vi "loadDTCs.vi"(10 "DTCs":T1[](array[typedef])) -> (2 "dtcs":string[](array[string]))   [LabVIEW 2018]
uses:
  <vilib>/Automotive Diagnostic Command Set/Diagnostic Protocols.llb/Diagnostic Trouble Code.ctl
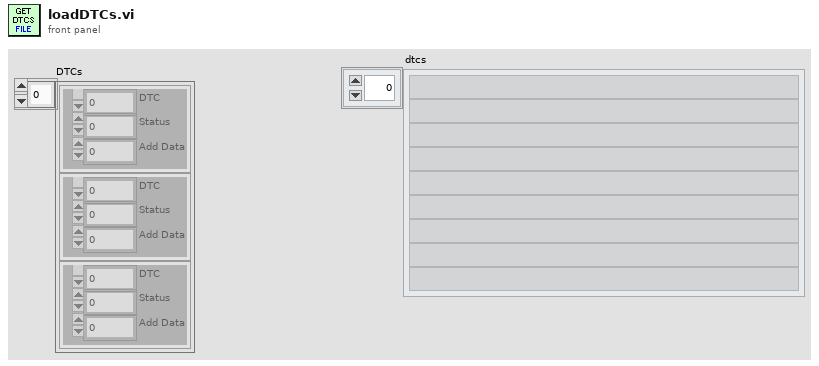
[diagram p1: front panel]
types:
  T1 = typedef "Diagnostic Trouble Code.ctl" = cluster{"DTC":u32, "Status":u32, "Add Data":u32}
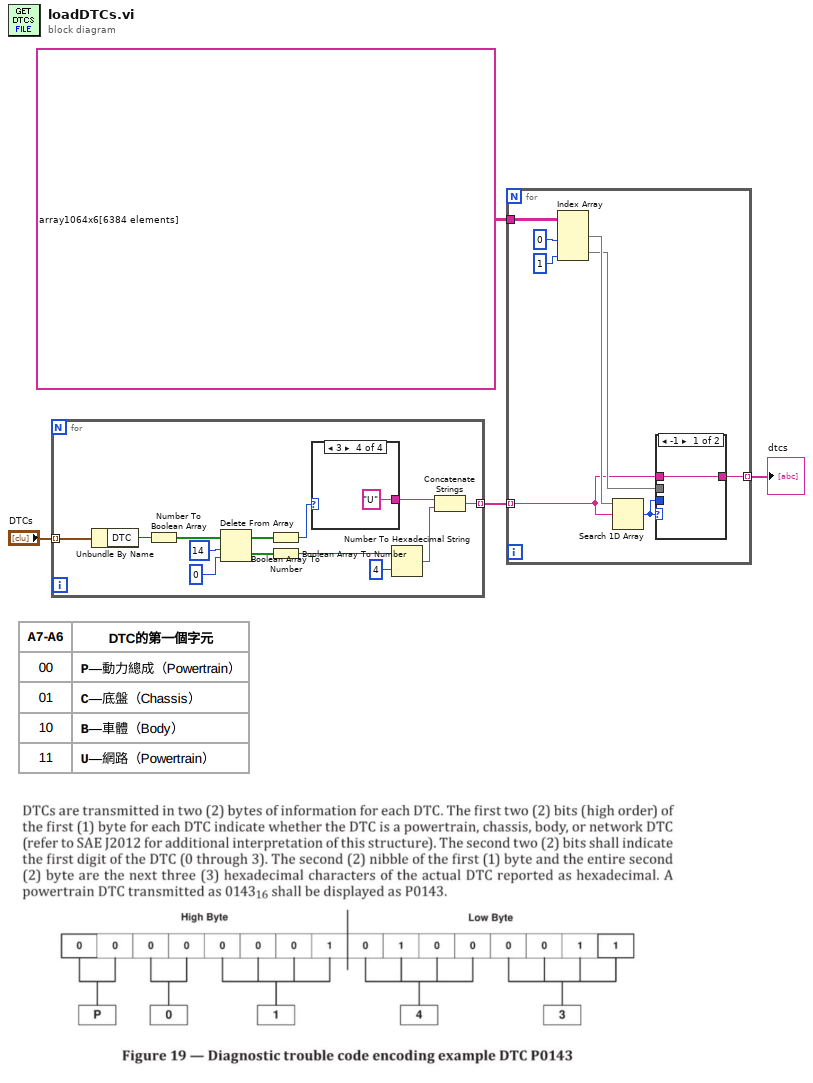
[diagram p0: block diagram]
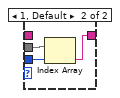
[diagram p2: hidden frame]
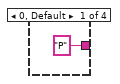
[diagram p3: hidden frame]
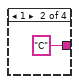
[diagram p4: hidden frame]
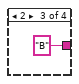
[diagram p5: hidden frame]
diagram:
  n1 = for {
    tunnel: "DTCs" -> [w17] mode=indexing
    tunnel: [w6] -> w2 mode=indexing
    n2 = Unbundle By Name(w17) -> ("DTC"=w16:u32)
    n3 = Number To Boolean Array(number=w16) -> (Boolean array=w15:bool[])
    n4 = Delete From Array(array=w15, length=14 ("长度"), index=0 ("索引")) -> (deleted portion=w11:bool[], array with subset deleted=w12:bool[])
    n5 = Boolean Array To Number(Boolean array=w12) -> (number=w9:u32)
    n6 = Boolean Array To Number(Boolean array=w11) -> (number=w10:u32)
    n7 = case shown="3" w9 {
      tunnel: ["P" "C" "B" "U"] -> w8
      frame 0, Default {
      }
      frame 1 {
      }
      frame 2 {
      }
      frame 3 {
      }
    }
    n8 = Number To Hexadecimal String(1:i16 4 ("宽度(-)"), 2:w10) -> (0:w7:string)
    n9 = Concatenate Strings(w8, w7) -> (w6:string)
  }
  n10 = for {
    tunnel: string[][] array1064x6[6384 elements] ("数组 2") -> [w29]
    tunnel: w2 -> [w23] mode=indexing
    tunnel: [w22] -> w1 mode=indexing
    n11 = Index Array(array=w29, index (col) #1=0 ("禁用的索引 (列)"), index (col) #2=1 ("索引 (列)")) -> (element #1=w26:string[], element #2=w25:string[])  [unwired: 2 in]
    n12 = Search 1D Array(1D array=w26, element=w23) -> (index of element=w24:i32)  [unwired: 1 in]
    n13 = case shown="-1" w24 {
      tunnel: w24 -> [_ w33]
      tunnel: w25 -> [_ w32]
      tunnel: [w30 w31] -> w22
      tunnel: w23 -> [w30 _]
      frame -1 {
      }
      frame 1, Default {
        n14 = Index Array(array=w32, index=w33) -> (element=w31:string)
      }
    }
  }
  "dtcs" <- w1
